vi "Serial Settings from ini.vi"(7 "Section":string, 8 "error in (no error)":errorcluster, 11 "Serial Port Settings In":T1={"VISA In"="COM1", "baud rate"=115200}) -> (0 "error out":errorcluster, 3 "Serial Port Settings Out":T1={"VISA In"="COM1", "baud rate"=115200}, 5 "All Tags Exists?":bool)   [LabVIEW 2013]
doc: "Loads the Serial settings from the ini file.\n\nPort - Com port number\nBaud Rate - configured speed. COM1 is maxed out at 115200"
uses:
  Common/File IO/INI/Read write mode.ctl
  Serial Enum Keys.ctl
  Serial/Serial Port Settings Cluster.ctl
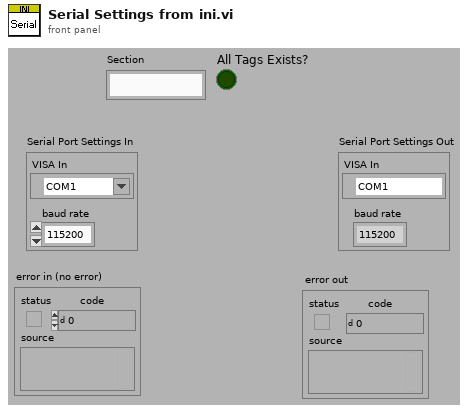
[diagram p1: front panel]
types:
  T1 = typedef "Serial Port Settings Cluster.ctl" = cluster{"VISA In":refnum<visa-resource-name>, "baud rate":u32}
  T2 = typedef "Serial Enum Keys.ctl" = enum16{"Port", "Baud Rate"}
  T3 = typedef "Read write mode.ctl" = enum16{"Read", "Write"}
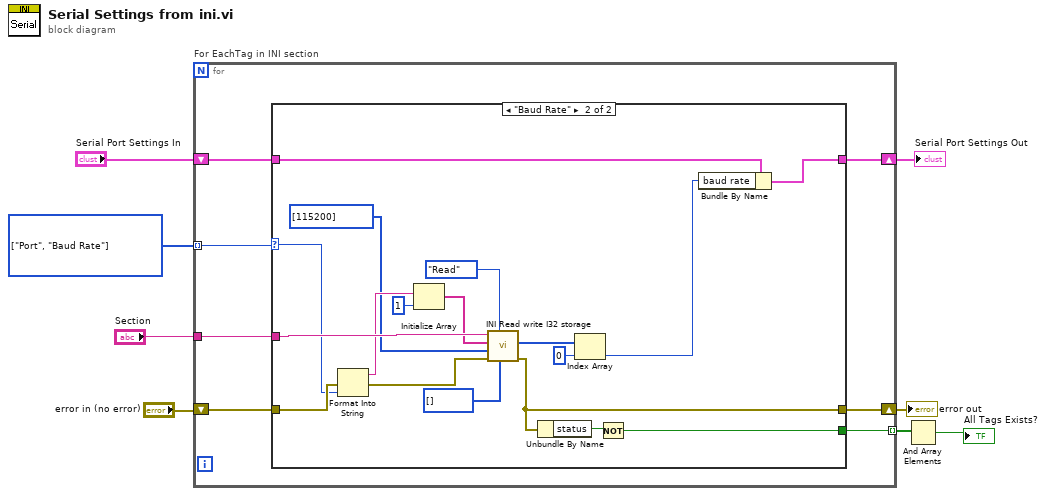
[diagram p0: block diagram]
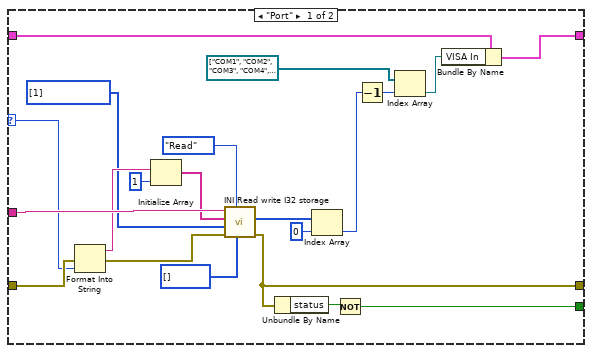
[diagram p2: hidden frame]
diagram:
  w8 = T2[] [enum."Port", enum."Baud Rate"] items=["Port", "Baud Rate"]
  n1 = for "For EachTag in INI section" {
    tunnel: "Section" -> [w15]
    tunnel: w8 -> [w14] mode=indexing
    shift-right: [w10] -> w6
    shift-left: "error in (no error)" -> [w12]
    shift-right: [w9] -> w1
    shift-left: "Serial Port Settings In" -> [w13]
    tunnel: [w11] -> w4 mode=indexing
    n2 = case shown="\"Baud Rate\"" w14 {
      selector: w14 -> [w31 w49]
      tunnel: w15 -> [w35 w53]
      tunnel: w13 -> [w33 w51]
      tunnel: w12 -> [w32 w50]
      tunnel: [w36 w54] -> w10
      tunnel: [w21 w39] -> w11
      tunnel: [w34 w52] -> w9
      frame "Port" {
        n3 = Format Into String(error in=w32, w31) -> (resulting string=w29:string, error out=w22:errorcluster)  [unwired: 2 in]
        n4 = Initialize Array(w29, 1 ("dimension size")) -> (w27:string[])
        n5 = call "INI Read write I32 storage.vi"("Values to write"=i32[] [], "Read/Write mode"=Read_write_mode."Read", "error in"=w22, "Defaults"=i32[] [1], "keys"=w27, "section"=w35) -> ("error out"=w36:errorcluster, "Values"=w26:i32[])  [unwired: 4 in]
        n6 = Unbundle By Name(w36) -> ("status"=w24:bool)
        n7 = Index Array(array=w26, index=0) -> (element=w19:i32)
        n8 = Not(x=w24) -> (.not. x?=w21:bool)
        n9 = Decrement(x=w19) -> (x-1=w17:i32)
        n10 = Index Array(array=refnum<visa-resource-name>[] ["COM1", "COM2", "COM3", "COM4", "COM5", "COM6", "COM7", "COM8", "COM9", "COM10", "COM11", "COM12", "COM13", "COM14", "COM15"], index=w17) -> (element=w16:refnum<visa-resource-name>)
        n11 = Bundle By Name(cluster=w33, "VISA In"=w16) -> (w34:T1)
      }
      frame "Baud Rate" {
        n12 = Format Into String(error in=w50, w49) -> (resulting string=w47:string, error out=w40:errorcluster)  [unwired: 2 in]
        n13 = Initialize Array(w47, 1 ("dimension size")) -> (w45:string[])
        n14 = call "INI Read write I32 storage.vi"("Values to write"=i32[] [], "Read/Write mode"=Read_write_mode."Read", "error in"=w40, "Defaults"=i32[] [115200], "keys"=w45, "section"=w53) -> ("error out"=w54:errorcluster, "Values"=w44:i32[])  [unwired: 4 in]
        n15 = Unbundle By Name(w54) -> ("status"=w42:bool)
        n16 = Index Array(array=w44, index=0) -> (element=w37:i32)
        n17 = Not(x=w42) -> (.not. x?=w39:bool)
        n18 = Bundle By Name(cluster=w51, "baud rate"=w37) -> (w52:T1)
      }
    }
  }
  "error out" <- w6
  "Serial Port Settings Out" <- w1
  n19 = And Array Elements(Boolean array=w4) -> (logical AND=→"All Tags Exists?":bool)
